vi "GEM_BANK_ARRAY_Size_if_Serialized.vi"(8 "error in (no error)":errorcluster, 11 "GEM_BANK_ARRAY in":refnum<class "GEM_BANK_ARRAY.lvclass">) -> (0 "error out":errorcluster, 2 "Size if Serialized":u32, 3 "GEM_BANK_ARRAY out":refnum<class "GEM_BANK_ARRAY.lvclass">)   [LabVIEW 2018, in "GEM_BANK_ARRAY.lvclass"]
uses:
  GEM_BANK_ARRAY.lvclass
  GEM_BANK_ARRAY.lvclass/GEM_BANK_ARRAY.ctl
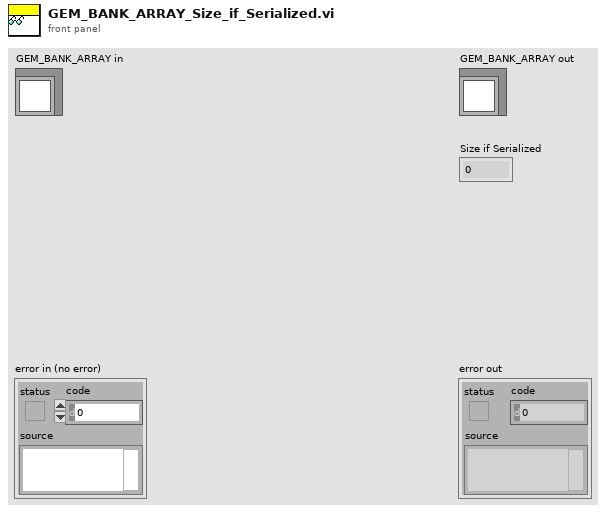
[diagram p1: front panel]
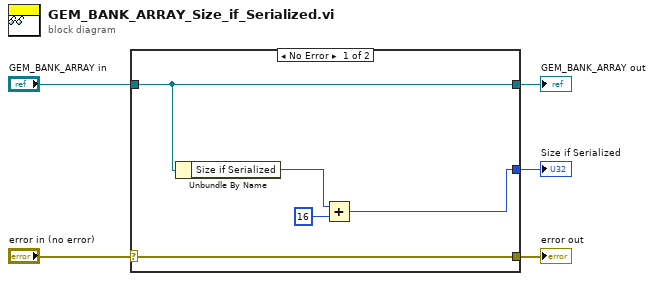
[diagram p0: block diagram]
diagram:
  n1 = case shown="No Error" "error in (no error)" {
    selector: "error in (no error)" -> [w10 w11]
    tunnel: [w10 w11] -> w4
    tunnel: [w9 w12] -> w2
    tunnel: "GEM_BANK_ARRAY in" -> [w9 w12]
    tunnel: [w6 _] -> w1
    frame No Error {
      n2 = Unbundle By Name(w9) -> ("Size if Serialized"=w8:u32)
      n3 = Add(x=w8, y=u32 16) -> (x+y=w6:u32)
    }
    frame Error {
    }
  }
  "error out" <- w4
  "GEM_BANK_ARRAY out" <- w2
  "Size if Serialized" <- w1
